vi "Write Client LNA Proxy.vi"(8 "error in (no error)":errorcluster, 10 "Actor Framework:Message Enqueuer":refnum<class "Message Enqueuer.lvclass">, 11 "Client Controller in":refnum<class "Client Controller.lvclass">) -> (0 "error out":errorcluster, 3 "Client Controller out":refnum<class "Client Controller.lvclass">)   [LabVIEW 2013, in "Client Controller.lvlib" / "Client Controller.lvclass"]
uses:
  Client Controller.lvclass
  <vilib>/ActorFramework/Message Enqueuer/Message Enqueuer.lvclass
  Client Controller.lvclass/Client Controller.ctl
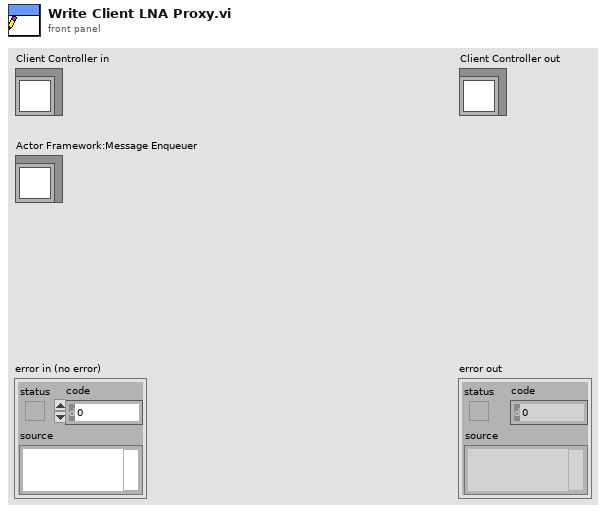
[diagram p1: front panel]
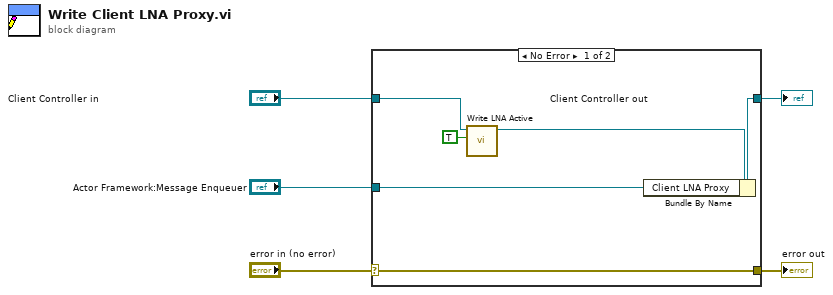
[diagram p0: block diagram]
diagram:
  n1 = case shown="No Error" "error in (no error)" {
    selector: "error in (no error)" -> [w11 w12]
    tunnel: [w11 w12] -> w4
    tunnel: [w10 w13] -> w2
    tunnel: "Client Controller in" -> [w8 w13]
    tunnel: "Actor Framework:Message Enqueuer" -> [w9 _]
    frame No Error {
      n2 = call "Write LNA Active.vi"("LNA Active?"=TRUE, "Client Controller in"=w8) -> ("Client Controller out"=w7:refnum<class "Client Controller.lvclass">)  [unwired: 8 in, 1 out]
      n3 = Bundle By Name(cluster=w7, "Client LNA Proxy"=w9) -> (w10:refnum<class "Client Controller.lvclass">)
    }
    frame Error {
    }
  }
  "error out" <- w4
  "Client Controller out" <- w2
